vi "Generate Workspace Velocity.vi"(8 "error in (no error)":errorcluster, 10 "workspace in":dbl[][](array[numeric]), 11 "Delta Analyzor in":refnum<class "Delta Analyzor.lvclass">) -> (0 "error out":errorcluster, 1 "velocities":dbl[][](array[numeric]), 2 "workspace out":dbl[][](array[numeric]), 3 "Delta Analyzor out":refnum<class "Delta Analyzor.lvclass">)   [LabVIEW 2013, in "Delta Analyzor.lvclass"]
uses:
  Delta Analyzor.lvclass
  Delta Analyzor.lvclass/Delta Analyzor.ctl
  Delta Robot Kinematics/Delta Robot Kinematics.lvclass
  <vilib>/Analysis/baseanly.llb/A x Vector.vi
  <vilib>/Analysis/NI_AALPro.lvlib
  <vilib>/Analysis/_algsub.llb/Real PseudoInverse Matrix.vi
  <vilib>/Analysis/NI_AALBase.lvlib
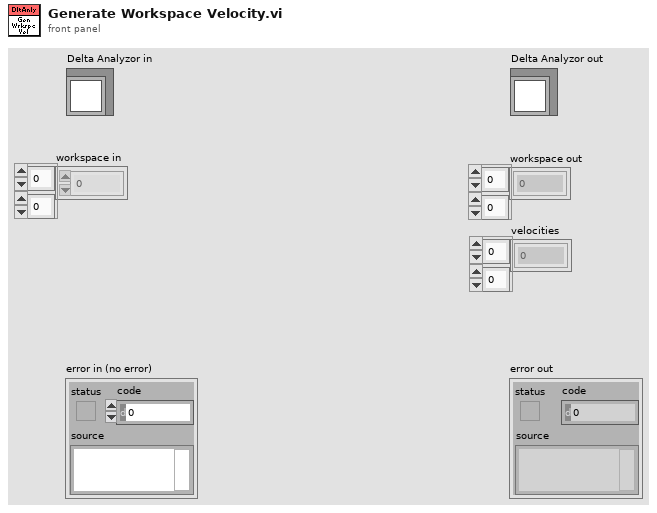
[diagram p1: front panel]
types:
  T1 = typedef "NI_Matrix.lvlib/RealMatrix.ctl" = dbl[][]
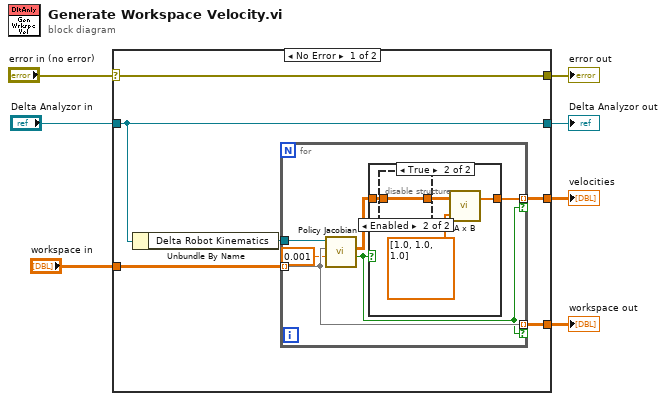
[diagram p0: block diagram]
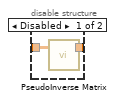
[diagram p3: hidden frame]
diagram:
  n1 = case shown="No Error" "error in (no error)" {
    selector: "error in (no error)" -> [w13 w28]
    tunnel: [w13 w28] -> w6
    tunnel: [w9 w27] -> w4
    tunnel: "Delta Analyzor in" -> [w9 w27]
    tunnel: "workspace in" -> [w12 _]
    tunnel: [w11 _] -> w2
    tunnel: [w10 _] -> w1
    frame No Error {
      n2 = Unbundle By Name(w9) -> ("Delta Robot Kinematics"=w8:refnum<class "Delta Robot Kinematics.lvclass">)
      n3 = for {
        tunnel: w12 -> [w17] mode=indexing
        tunnel: [w18] -> w10 mode=indexing if=w16
        tunnel: [w17] -> w11 mode=indexing if=w16
        tunnel: w8 -> [w15]
        n4 = call-dynamic "Policy Jacobian.vi"("delta"=0.001, "ref p"=w17, "Delta Robot Kinematics in"=w15) -> ("calulated"=w16:bool, "Jacobian"=w19:T1)  [unwired: 5 in, 2 out]
        n5 = case shown="True" w16 {
          tunnel: w19 -> [_ w23]
          tunnel: [_ w20] -> w18
          frame False {
          }
          frame True {
            n6 = disable-structure shown="Enabled" {
              disable-tunnel: w23 -> [w25 w26]
              disable-tunnel: [w24 w26] -> w22
              frame Disabled {
                n7 = call-poly <vilib>:"PseudoInverse Matrix.vi"("Input Matrix"=w25) -> ("PseudoInverse Matrix"=w24:T1)  [unwired: 1 in, 1 out]
              }
              frame Enabled {
              }
            }
            n8 = call-poly <vilib>:"A x B.vi"("Vector"=dbl[] [1.0, 1.0, 1.0], "A"=w22) -> ("A x Vector"=w20:dbl[])  [unwired: 1 out]
          }
        }
      }
    }
    frame Error {
    }
  }
  "error out" <- w6
  "Delta Analyzor out" <- w4
  "velocities" <- w1
  "workspace out" <- w2
